vi "Day 17-1.vi"() -> ()   [LabVIEW 2020]
uses:
  Probe Target.ctl
  Probe.ctl
panel:
  out "x-y":dbl
  out "Array":T1[](array[typedef])
  in  "dY Min":i32=-102
  out "Count":i32
  in  "dY Max":i32=101
  in  "dX Max":i32=155
  out "XY Graph":cluster{i32, i32}[](graph)
  in  "Probe":T1
  in  "Probe Target":T2={"X Min"=135, "X Max"=155, "Y Min"=-102, "Y Max"=-78}
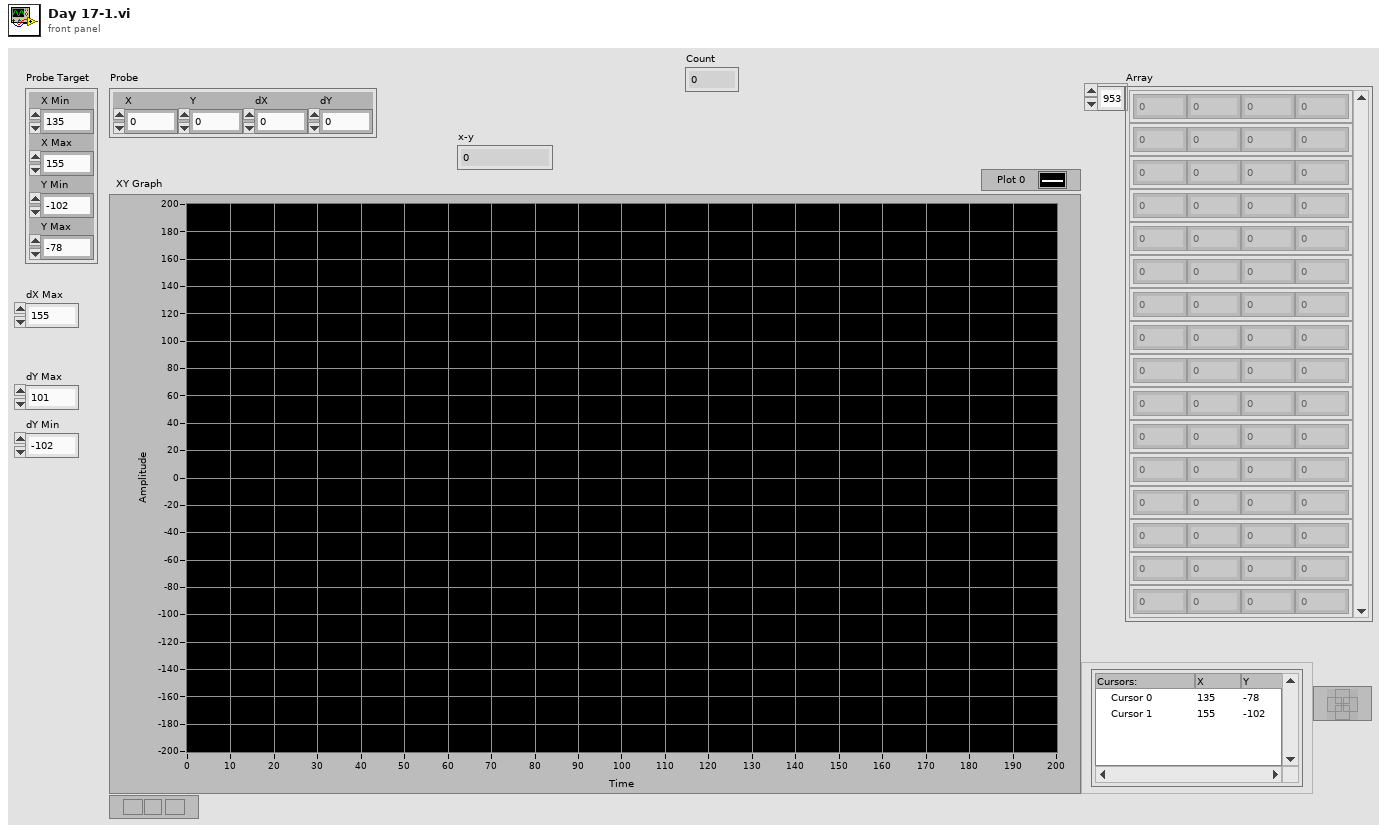
[diagram p1: front panel]
types:
  T1 = typedef "Probe.ctl" = cluster{"X":i32, "Y":i32, "dX":i32, "dY":i32}
  T2 = typedef "Probe Target.ctl" = cluster{"X Min":i32, "X Max":i32, "Y Min":i32, "Y Max":i32}
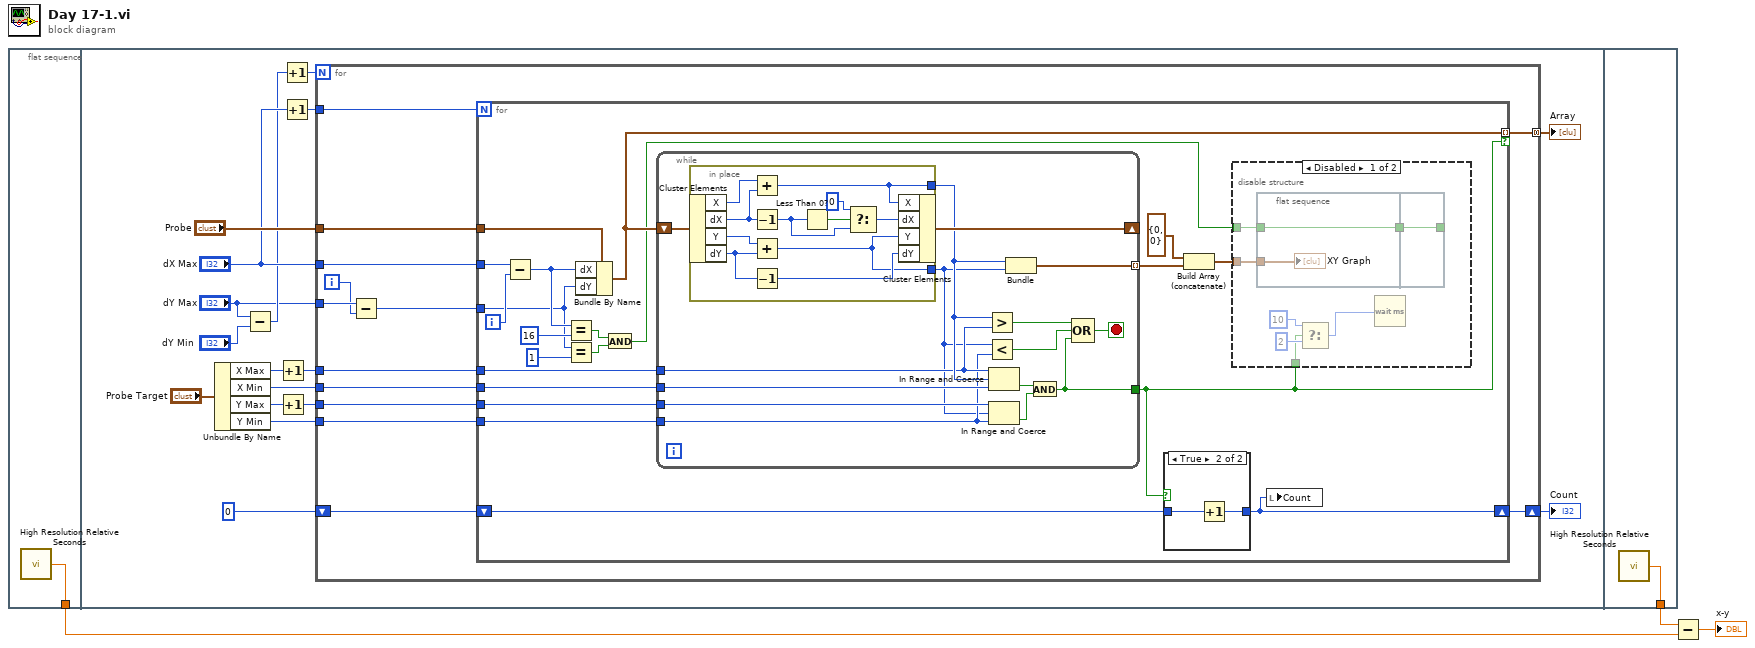
[diagram p0: block diagram]
diagram:
  n1 = flat-sequence {
    tunnel: [w4] -> w2
    tunnel: [w95] -> w3
    frame #0 {
      n2 = call <vilib>:"High Resolution Relative Seconds.vi"() -> ("relative seconds"=w4:dbl)
    }
    frame #1 {
      n3 = Unbundle By Name("Probe Target") -> ("X Max"=w17:i32, "X Min"=w19:i32, "Y Max"=w18:i32, "Y Min"=w14:i32)
      n4 = Subtract(x="dY Max", y="dY Min") -> (x-y=w9:i32)
      n5 = Increment(x=w17) -> (x+1=w16:i32)
      n6 = Increment(x=w18) -> (x+1=w15:i32)
      n7 = Increment(x=w9) -> (x+1=w6:i32)
      n8 = Increment(x="dX Max") -> (x+1=w5:i32)
      n9 = for {
        N: w6 -> [_]
        tunnel: "Probe" -> [w34]
        tunnel: w19 -> [w33]
        tunnel: w16 -> [w32]
        tunnel: w15 -> [w31]
        tunnel: w14 -> [w30]
        tunnel: "dX Max" -> [w23]
        shift-right: [w28] -> w11
        shift-left: 0 -> [w29]
        tunnel: w5 -> [w27]
        tunnel: "dY Max" -> [w25]
        tunnel: [w26] -> w7 mode=concatenating
        i -> [w24]
        n10 = Subtract(x=w25, y=w24) -> (x-y=w22:i32)
        n11 = for {
          N: w27 -> [_]
          tunnel: w34 -> [w55]
          tunnel: w33 -> [w54]
          tunnel: w32 -> [w53]
          tunnel: w31 -> [w52]
          tunnel: w30 -> [w51]
          shift-right: [w35] -> w28
          shift-left: w29 -> [w50]
          tunnel: [w48] -> w26 mode=indexing if=w36
          tunnel: w23 -> [w40]
          tunnel: w22 -> [w37]
          i -> [w39]
          n12 = Subtract(x=w40, y=w39) -> (x-y=w38:i32)
          n13 = Equal?(x=w38, y=16) -> (x = y?=w43:bool)
          n14 = Equal?(x=w37, y=1) -> (x = y?=w42:bool)
          n15 = Bundle By Name(cluster=w55, "dX"=w38, "dY"=w37) -> (w48:T1)
          n16 = And(x=w43, y=w42) -> (x .and. y?=w41:bool)
          n17 = while {
            shift-right: [w82] -> _
            shift-left: w48 -> [w83]
            tunnel: w54 -> [w80]
            tunnel: [w81] -> w49 mode=indexing
            tunnel: w52 -> [w79]
            tunnel: w53 -> [w73]
            tunnel: w51 -> [w71]
            tunnel: [w75] -> w36
            stop <- w76 stop-if-true
            n18 = in-place {
              in-place-border: [w85] -> w69
              in-place-border: [w84] -> w74
              n19 = in-place-cluster #1(w83) -> ("X"=w94:i32, "dX"=w93:i32, "Y"=w88:i32, "dY"=w87:i32)
              n20 = Add(x=w94, y=w93) -> (x+y=w84:i32)
              n21 = Decrement(x=w93) -> (x-1=w91:i32)
              n22 = Add(x=w88, y=w87) -> (x+y=w85:i32)
              n23 = Decrement(x=w87) -> (x-1=w86:i32)
              n24 = Less Than 0?(x=w91) -> (x < 0?=w92:bool)
              n25 = Select(t=0, s=w92, f=w91) -> (s? t:f=w89:i32)
              n26 = in-place-cluster #1("X"=w84, "dX"=w89, "Y"=w85, "dY"=w86) -> (w82:T1)
            }
            n27 = Greater?(x=w74, y=w73) -> (0:w72:bool)
            n28 = Less?(x=w69, y=w71) -> (x < y?=w70:bool)
            n29 = In Range and Coerce(upper limit=w73, x=w74, lower limit=w80) -> (In Range?=w78:bool)  [unwired: 1 out]
            n30 = In Range and Coerce(upper limit=w79, x=w69, lower limit=w71) -> (In Range?=w77:bool)  [unwired: 1 out]
            n31 = Bundle(w74, w69) -> (w81:cluster{i32, i32})  [unwired: 1 in]
            n32 = And(x=w78, y=w77) -> (x .and. y?=w75:bool)
            n33 = Compound Arithmetic op=OR(w72, w70, w75) -> (w76:bool)
          }
          n34 = case shown="True" w36 {
            tunnel: w50 -> [w66 w68]
            tunnel: [w66 w67] -> w35
            frame False {
            }
            frame True {
              n35 = Increment(x=w68) -> (x+1=w67:i32)
            }
          }
          n36 = Build Array (concatenate)(cluster{i32, i32} {0, 0} ("output cluster"), w49) -> (w47:cluster{i32, i32}[])
          n37 = disable-structure shown="Disabled" {
            disable-tunnel: w47 -> [w61 _]
            disable-tunnel: w41 -> [w60 _]
            disable-tunnel: w36 -> [w57 _]
            frame Disabled {
              n38 = flat-sequence {
                tunnel: w61 -> [w64]
                tunnel: w60 -> [w63]
                tunnel: [w63] -> w62
                tunnel: [w65] -> _
                tunnel: w62 -> [w65]
                frame #0 {
                  "XY Graph" <- w64
                }
                frame #1 {
                }
              }
              n39 = Select(t=u32 10 ("milliseconds to wait"), s=w57, f=u32 2 ("milliseconds to wait")) -> (s? t:f=w56:u32)
              n40 = Wait (ms)(milliseconds to wait=w56) -> ()  [unwired: 1 out]
            }
            frame Enabled {
            }
          }
          n41 = local write "Count"(w35) -> ()
        }
      }
      "Count" <- w11
      "Array" <- w7
    }
    frame #2 {
      n42 = call <vilib>:"High Resolution Relative Seconds.vi"() -> ("relative seconds"=w95:dbl)
    }
  }
  n43 = Subtract(x=w3, y=w2) -> (x-y=→"x-y":dbl)
